vi "pump calibration dialog.vi"() -> ()   [LabVIEW 2015]
uses:
  calibration commands.ctl
panel:
  in  "Test High rpm":bool
  in  "Test Low rpm":bool
  in  "pump ID":u8
  in  "RPM Calibration":T1={"target 1"=10.0, "target 2"=90.0, "measured 1"=0.0, "measured 2"=0.0}
  in  "STAMP intercept":dbl
  in  "STAMP slope":dbl=1.0
  in  "OK Button":bool
  # "To calibrate pump rpm to match the speed that is being sent from ProCoDA\n\n1) Make sure the pump is turned on and is running. The set rpm doesn't matter here.\n2) Select correct Pump ID\n3) Enter a low and a high target speed (normally use 10 and 90 as percent of full speed)\n4) Test Low rpm and enter the measured rpm using the digital pump display.\n5) Test High rpm and enter the measured rpm using the digital pump display.\n6) The pump should immediately return to the correct rpm that is set by ProCoDA\nThese steps will set 600 rpm pumps so that they run 100 rpm when sent a ProCoDA value of 1 \n\nTo calibrate flow rate continue with these steps.\n7) Set the pump control to 0.5 for 100 rpm pumps or 3 for 600 rpm pumps.\n8) While it is running, use either a bucket and stopwatch or a balance to measure the flow rate from the pump.\n9) After you have collected enough data to have a confident value for the flow rate, stop the pump.\n10) Calculate the actual mL/rev value for your tubing by dividing the flow rate by the pump rpm.\n11) For the set point where you have recorded the factory value of mL/rev for your tubing, replace its value with the value calculated in step 10."
  # "Set the pump ID first!"
  # "rpm"
  # "rpm"
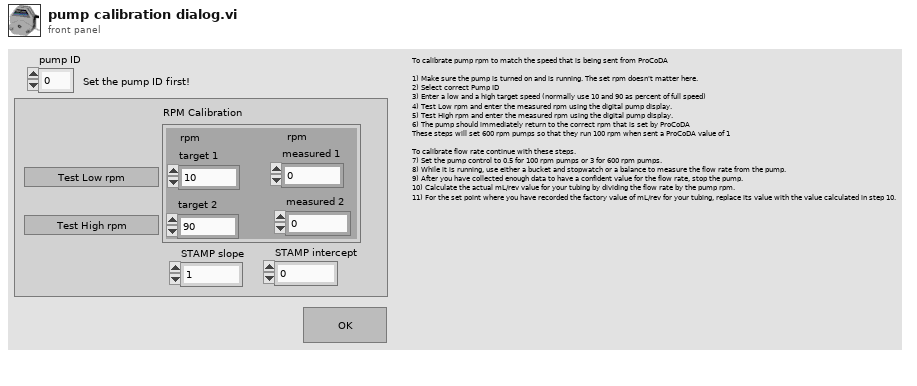
[diagram p1: front panel]
types:
  T1 = cluster{"target 1":dbl, "target 2":dbl, "measured 1":dbl, "measured 2":dbl}
  T2 = typedef "calibration commands.ctl" = enum16{"Get ini Path", "Save default values", "Save new calibration", "Read calibration", "Apply calibration", "Read STAMP mb", "Write STAMP mb"}
  T3 = typedef "calibration values.ctl" = cluster{"target 1":dbl[unit], "target 2":dbl[unit], "measured 1":dbl[unit], "measured 2":dbl[unit]}
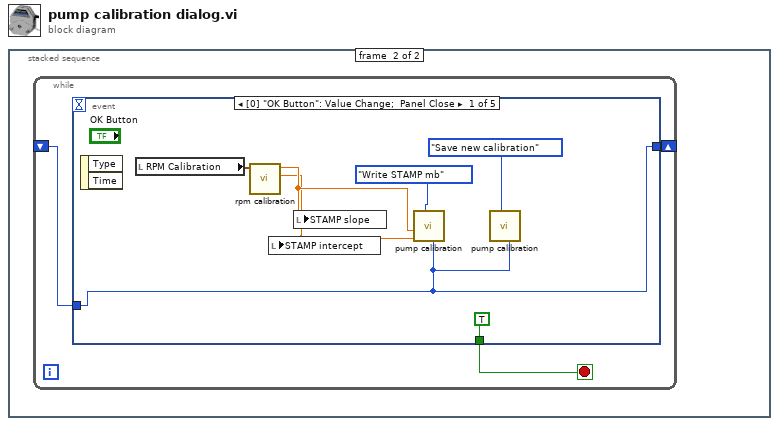
[diagram p0: block diagram]
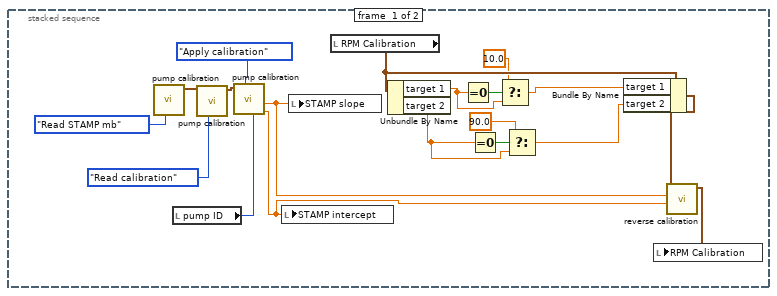
[diagram p2: hidden frame]
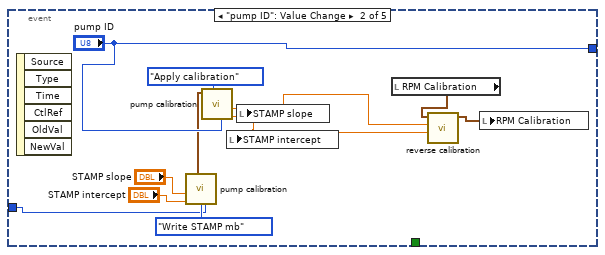
[diagram p3: hidden frame]
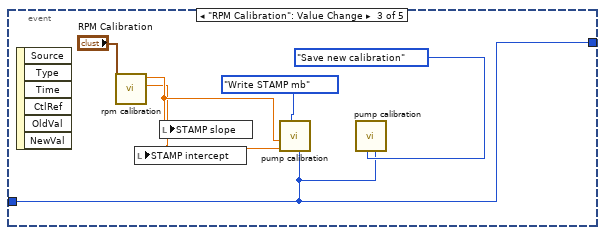
[diagram p4: hidden frame]
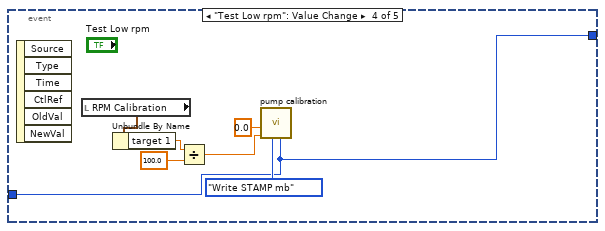
[diagram p5: hidden frame]
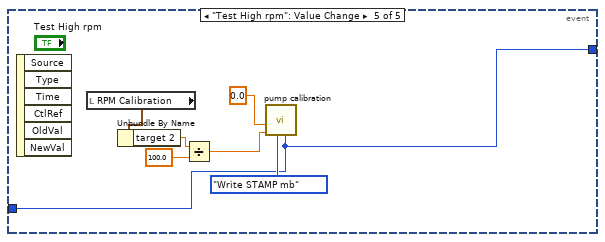
[diagram p6: hidden frame]
diagram:
  n1 = stacked-sequence {
    frame #0 {
      n2 = call "pump calibration.vi"("pump cal command"=calibration_commands."Read STAMP mb") -> ("Pump Calibration out"=w16:T3)  [unwired: 7 in, 3 out]
      n3 = local read "pump ID"() -> (w18:u8)
      n4 = call "pump calibration.vi"("pump cal command"=calibration_commands."Read calibration", "Pump Calibration in"=w16) -> ("Pump Calibration out"=w15:T3)  [unwired: 6 in, 3 out]
      n5 = call "pump calibration.vi"("pump ID"=w18, "pump cal command"=calibration_commands."Apply calibration", "Pump Calibration in"=w15) -> ("STAMP intercept out"=w11:dbl, "STAMP slope out"=w12:dbl)  [unwired: 5 in, 2 out]
      n6 = local write "STAMP intercept"(w11) -> ()
      n7 = local write "STAMP slope"(w12) -> ()
      n8 = local read "RPM Calibration"() -> (w10:T1)
      n9 = Unbundle By Name(w10) -> ("target 1"=w7:dbl, "target 2"=w3:dbl)
      n10 = Equal To 0?(x=w7) -> (x = 0?=w8:bool)
      n11 = Equal To 0?(x=w3) -> (x = 0?=w4:bool)
      n12 = Select(t=10.0, s=w8, f=w7) -> (s? t:f=w6:dbl)
      n13 = Select(t=90.0, s=w4, f=w3) -> (s? t:f=w1:dbl)
      n14 = Bundle By Name(cluster=w10, "target 1"=w6, "target 2"=w1) -> (w9:T1)
      n15 = call "reverse calibration.vi"("STAMP intercept"=w11, "STAMP slope"=w12, "RPM Calibration in"=w9) -> ("RPM Calibration"=w13:T1)  [unwired: 8 in]
      n16 = local write "RPM Calibration"(w13) -> ()
    }
    frame #1 {
      n17 = while {
        shift-right: [w21] -> _
        shift-left: _ -> [w20]
        stop <- w22 stop-if-true
        n18 = event shown="[0] \"OK Button\": Value Change;  Panel Close" {
          selector: _ -> [_ _ _ _ _]
          dyn-events: _ -> [_ _ _ _ _]
          timeout: _ -> [_ _ _ _ _]
          tunnel: [TRUE _ _ _ _] -> w22
          tunnel: [w23 "pump ID" w42 w47 w54] -> w21
          tunnel: w20 -> [w23 w37 w42 w47 w54]
          event "OK Button": Value Change; Panel Close {
            n19 = event-data() -> ()  [unwired: 1 in, 2 out]
            n20 = local read "RPM Calibration"() -> (w28:T1)
            n21 = call "rpm calibration.vi"("RPM Calibration"=w28) -> ("STAMP intercept"=w26:dbl, "STAMP slope"=w27:dbl)  [unwired: 9 in]
            n22 = local write "STAMP intercept"(w26) -> ()
            n23 = local write "STAMP slope"(w27) -> ()
            n24 = call "pump calibration.vi"("pump ID"=w23, "pump cal command"=calibration_commands."Write STAMP mb", "STAMP intercept"=w26, "STAMP slope"=w27) -> ()  [unwired: 4 in, 4 out]
            n25 = call "pump calibration.vi"("pump ID"=w23, "pump cal command"=calibration_commands."Save new calibration") -> ()  [unwired: 6 in, 4 out]
          }
          event "pump ID": Value Change {
            n26 = event-data() -> ()  [unwired: 1 in, 6 out]
            n27 = call "pump calibration.vi"("pump ID"=w37, "pump cal command"=calibration_commands."Write STAMP mb", "STAMP intercept"="STAMP intercept", "STAMP slope"="STAMP slope") -> ("Pump Calibration out"=w36:T3)  [unwired: 4 in, 3 out]
            n28 = call "pump calibration.vi"("pump ID"="pump ID", "pump cal command"=calibration_commands."Apply calibration", "Pump Calibration in"=w36) -> ("STAMP intercept out"=w32:dbl, "STAMP slope out"=w33:dbl)  [unwired: 5 in, 2 out]
            n29 = local write "STAMP intercept"(w32) -> ()
            n30 = local write "STAMP slope"(w33) -> ()
            n31 = local read "RPM Calibration"() -> (w30:T1)
            n32 = call "reverse calibration.vi"("STAMP intercept"=w32, "STAMP slope"=w33, "RPM Calibration in"=w30) -> ("RPM Calibration"=w31:T1)  [unwired: 8 in]
            n33 = local write "RPM Calibration"(w31) -> ()
          }
          event "RPM Calibration": Value Change {
            n34 = event-data() -> ()  [unwired: 1 in, 6 out]
            n35 = call "rpm calibration.vi"("RPM Calibration"="RPM Calibration") -> ("STAMP intercept"=w45:dbl, "STAMP slope"=w46:dbl)  [unwired: 9 in]
            n36 = local write "STAMP intercept"(w45) -> ()
            n37 = local write "STAMP slope"(w46) -> ()
            n38 = call "pump calibration.vi"("pump ID"=w42, "pump cal command"=calibration_commands."Write STAMP mb", "STAMP intercept"=w45, "STAMP slope"=w46) -> ()  [unwired: 4 in, 4 out]
            n39 = call "pump calibration.vi"("pump ID"=w42, "pump cal command"=calibration_commands."Save new calibration") -> ()  [unwired: 6 in, 4 out]
          }
          event "Test Low rpm": Value Change {
            n40 = event-data() -> ()  [unwired: 1 in, 6 out]
            n41 = local read "RPM Calibration"() -> (w53:T1)
            n42 = Unbundle By Name(w53) -> ("target 1"=w52:dbl)
            n43 = Divide(x=w52, y=100.0) -> (x/y=w49:dbl)
            n44 = call "pump calibration.vi"("pump ID"=w47, "pump cal command"=calibration_commands."Write STAMP mb", "STAMP intercept"=w49, "STAMP slope"=0.0) -> ()  [unwired: 4 in, 4 out]
          }
          event "Test High rpm": Value Change {
            n45 = event-data() -> ()  [unwired: 1 in, 6 out]
            n46 = local read "RPM Calibration"() -> (w60:T1)
            n47 = Unbundle By Name(w60) -> ("target 2"=w59:dbl)
            n48 = Divide(x=w59, y=100.0) -> (x/y=w55:dbl)
            n49 = call "pump calibration.vi"("pump ID"=w54, "pump cal command"=calibration_commands."Write STAMP mb", "STAMP intercept"=w55, "STAMP slope"=0.0) -> ()  [unwired: 4 in, 4 out]
          }
        }
      }
    }
  }
